vi "Write configuration.vi"(8 "error in (no error)":errorcluster, 10 "configuration":string, 11 "Start in":refnum<class "Start.lvclass">) -> (0 "error out":errorcluster, 3 "Start out":refnum<class "Start.lvclass">)   [LabVIEW 2016, in "Commands.lvlib" / "Start.lvclass"]
uses:
  Start.lvclass
  Start.lvclass/Start.ctl
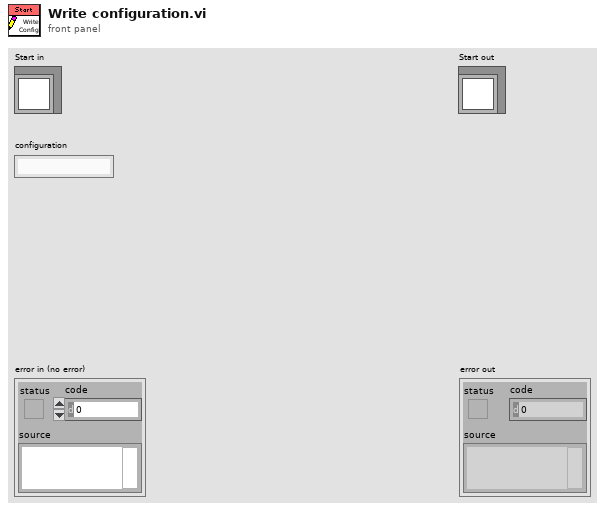
[diagram p1: front panel]
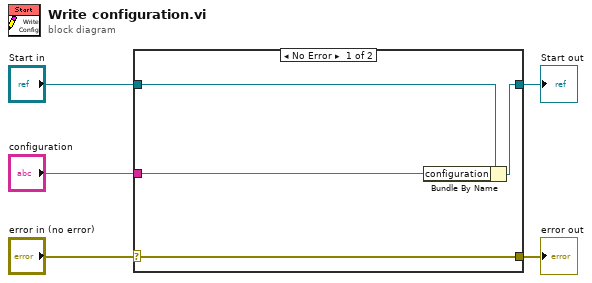
[diagram p0: block diagram]
diagram:
  n1 = case shown="No Error" "error in (no error)" {
    selector: "error in (no error)" -> [w9 w10]
    tunnel: [w9 w10] -> w4
    tunnel: [w7 w11] -> w2
    tunnel: "Start in" -> [w8 w11]
    tunnel: "configuration" -> [w6 _]
    frame No Error {
      n2 = Bundle By Name(cluster=w8, "configuration"=w6) -> (w7:refnum<class "Start.lvclass">)
    }
    frame Error {
    }
  }
  "error out" <- w4
  "Start out" <- w2
